vi "Auto Setup.vi"(8 "error in":errorcluster) -> (0 "error out":errorcluster)   [LabVIEW 2020]
uses:
  <vilib>/Rock Robotics/WPI/DriverStation/WPI_DriverStationRobotMode2.ctl
  b3a484b6-3d34-4235-842a-44c07264b682.vi
  19e807a5-ee4b-41d9-ac37-e9a2df102fa4.vi
  Framework/Robot Global Data.vi
  <vilib>/Rock Robotics/Network Tables/NT Write String Array.vi
  <vilib>/Rock Robotics/Network Tables/NT Write Variant.vi
  <vilib>/Rock Robotics/Network Tables/NT Read String.vi
panel:
  in  "override":bool=TRUE
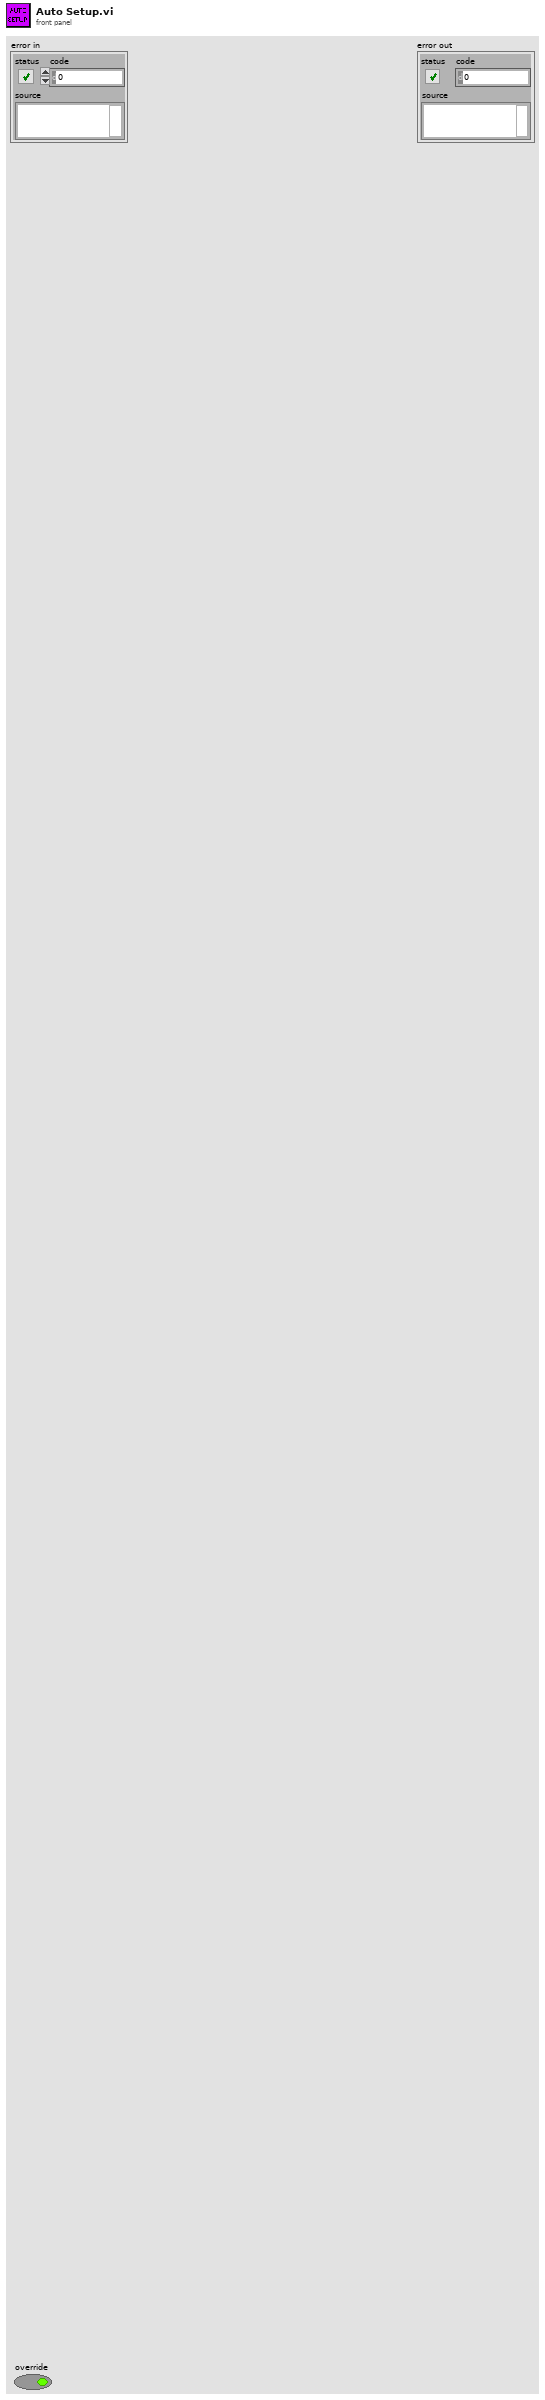
[diagram p1: front panel]
types:
  T1 = typedef "WPI_DriverStationRobotMode2.ctl" = enum16{"Autonomous Disabled", "Autonomous Enabled", "Teleop Disabled", "Teleop Enabled", "Disconnected", "Finish", "Test Disabled", "Test Enabled", "Emergency Stopped"}
  T2 = cluster{"Robot Backwards":bool, "Reverse Path":bool}
  T3 = cluster{"Segment Name":string, "Type":enum16{"Accel Straight", "Const Straight", "Blend", "Circle"}, "Traj Pos Points":cluster{"x":dbl, "y":dbl, "th":dbl}[], "Traj Vel Points":cluster{"V":dbl, "th":dbl}[], "Accel Index":i32, "Decel Index":i32}[]
  T4 = typedef "Single Cmd Info.ctl" = cluster{"Name":string, "CPTM.DataType":variant, "All Control Values Variant":cluster{"Name":string, "Variant Data":variant}[], "icon full":T5, "icon scaled":T5, "Path":path, "Subsystem Color":u32}
  T5 = typedef "imagedata.ctl" = cluster{"image type":i32, "image depth":i32, "image":u8[], "mask":u8[], "colors":u32[], "Rectangle":cluster{"left":i16, "top":i16, "right":i16, "bottom":i16}}
  T6 = typedef "Overrides.ctl" = cluster{"Count":string, "Angular Override":dbl, "Enabled?":bool, "Velocity Override":dbl, "Angle Override":dbl}[]
  T7 = typedef "Angluar Limits.ctl" = cluster{"Velocity (deg/s)":dbl, "Accel (deg/s^2)":dbl, "Jerk (deg/s^3)":dbl}
  T8 = cluster{"Sample Period (s)":dbl, cluster{"Velocity (fps)":dbl, "Accel (fps^2)":dbl, "Jerk (fps^3)":dbl, "StoopidFast (fps)":dbl}, "Conditions":cluster{"vInitial (fps)":dbl, "vFinal (fps)":dbl}, "Overrides":T6, "Angular Limits":T7}
  T9 = typedef "Drive Type.ctl" = enum16{"Nonholonomic", "Holonomic"}
  T10 = typedef "Path Type.ctl" = enum16{"Clothoid", "Bezier"}
  T11 = cluster{"Overall":cluster{"Time (s)":dbl, "Distance (ft)":dbl}, "Points out":cluster{"x":dbl, "y":dbl, "th":dbl}[], "Commands out":cluster{"Time (s)":dbl, T4, bool}[], "Zero V":bool, "Trajectory Data":cluster{"Segment Name":string, "Type":enum16{"Accel Straight", "Const Straight", "Blend", "Circle"}, "Traj Pos Points":cluster{"x":dbl, "y":dbl, "th":dbl}[], "Traj Vel Points":cluster{"V":dbl, "th":dbl}[], "Accel Index":i32, "Decel Index":i32}[], "Reversals":cluster{"Robot Backwards":bool, "Reverse Path":bool}, "Fields":cluster{"Sample Period (s)":dbl, cluster{"Velocity (fps)":dbl, "Accel (fps^2)":dbl, "Jerk (fps^3)":dbl, "StoopidFast (fps)":dbl}, "Conditions":cluster{"vInitial (fps)":dbl, "vFinal (fps)":dbl}, "Overrides":T6, "Angular Limits":T7}, "Trajectory Meta":cluster{"Drive Type":T9, "Path Type":T10}}
  T12 = cluster{"Traj Vel Points":cluster{"V":dbl, "th":dbl}[], "Reversals":cluster{"Robot Backwards":bool, "Reverse Path":bool}}
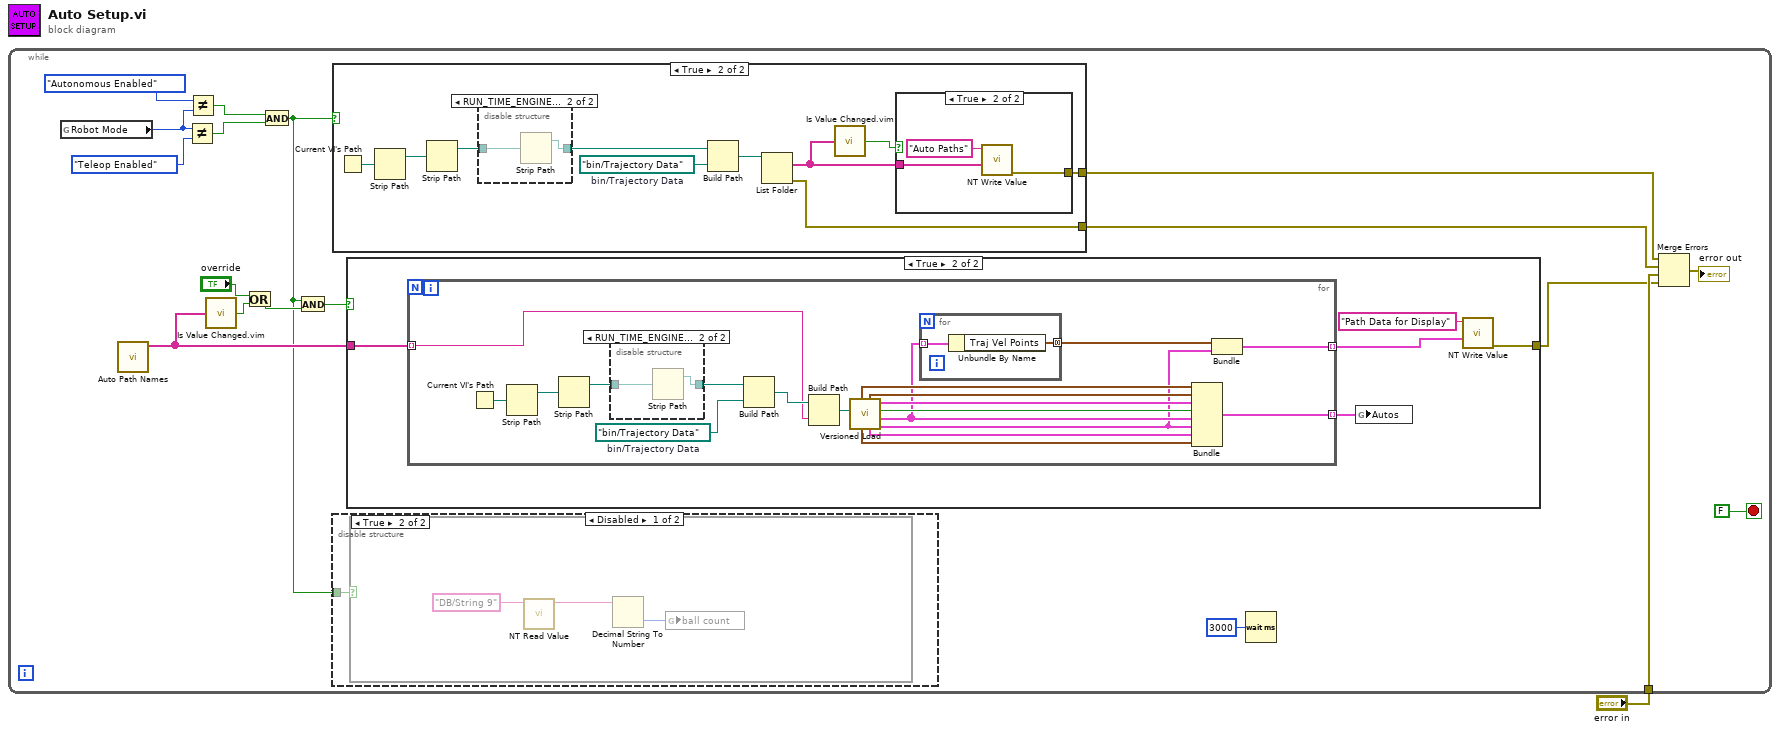
[diagram p0: block diagram]
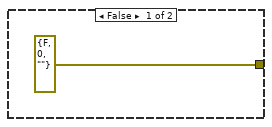
[diagram p4: hidden frame]
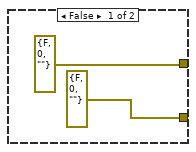
[diagram p6: hidden frame]
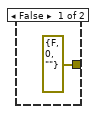
[diagram p7: hidden frame]
diagram:
  n1 = while {
    tunnel: "error in" -> [w3]
    stop <- FALSE stop-if-true
    n2 = global read "Robot Global Data.vi" "Robot Mode"() -> (w17:T1)
    n3 = call "Auto Path Names.vi"() -> ("Path Names"=w5:string[])  [unwired: 11 in]
    n4 = Not Equal?(x=w17, y=WPI_DriverStationRobotMode2."Teleop Enabled") -> (x != y?=w14:bool)
    n5 = Not Equal?(x=WPI_DriverStationRobotMode2."Autonomous Enabled", y=w17) -> (x != y?=w15:bool)
    n6 = call "Is Value Changed.vim"("value"=w5) -> ("changed or first call?"=w8:bool)
    n7 = Or(x="override", y=w8) -> (x .or. y?=w6:bool)
    n8 = And(x=w15, y=w14) -> (x .and. y?=w4:bool)
    n9 = And(x=w4, y=w6) -> (x .and. y?=w13:bool)
    n10 = case shown="True" w4 {
      tunnel: [errorcluster {"status"=FALSE, "code"=0, "source"=""} ("error out") w59] -> w12
      tunnel: [errorcluster {"status"=FALSE, "code"=0, "source"=""} ("error out") w58] -> w10
      frame False {
      }
      frame True {
        w60 = path "bin/Trajectory Data"  # bin/Trajectory Data
        n11 = Current VI's Path() -> (path=w61:path)
        n12 = Strip Path(path=w61) -> (stripped path=w62:path)  [unwired: 1 out]
        n13 = Strip Path(path=w62) -> (stripped path=w64:path)  [unwired: 1 out]
        n14 = disable-structure shown="RUN_TIME_ENGINE==True, Default" {
          disable-tunnel: [w70 w71] -> w63
          disable-tunnel: w64 -> [w70 w72]
          frame condition #0 (active) {
          }
          frame condition #1 {
            n15 = Strip Path(path=w72) -> (stripped path=w71:path)  [unwired: 1 out]
          }
        }
        n16 = Build Path(base path=w63, name or relative path=w60) -> (appended path=w65:path)
        n17 = List Folder(path=w65) -> (filenames=w57:string[], error out=w59:errorcluster)  [unwired: 3 in, 2 out]
        n18 = call "Is Value Changed.vim"("value"=w57) -> ("changed or first call?"=w56:bool)
        n19 = case shown="True" w56 {
          tunnel: w57 -> [_ w68]
          tunnel: [errorcluster {"status"=FALSE, "code"=0, "source"=""} ("error out") w67] -> w58
          frame False {
          }
          frame True {
            n20 = call-poly <vilib>:"NT Write Value.vi"("String Array"=w68, "Name"="Auto Paths") -> ("error out"=w67:errorcluster)  [unwired: 9 in]
          }
        }
      }
    }
    n21 = disable-structure shown="Disabled" {
      disable-tunnel: w4 -> [w20 _]
      frame Disabled {
        n22 = case shown="True" w20 {
          frame False {
          }
          frame True {
            n23 = call-poly <vilib>:"NT Read Value.vi"("Name"="DB/String 9") -> ("String"=w22:string)  [unwired: 9 in, 1 out]
            n24 = Decimal String To Number(string=w22) -> (number=w21:i32)  [unwired: 2 in, 1 out]
            n25 = global write "Robot Global Data.vi" "ball count"(w21) -> ()
          }
        }
      }
      frame Enabled {
      }
    }
    n26 = case shown="True" w13 {
      tunnel: w5 -> [_ w27]
      tunnel: [errorcluster {"status"=FALSE, "code"=0, "source"=""} ("error out") w28] -> w2
      frame False {
      }
      frame True {
        n27 = for {
          tunnel: w27 -> [w42] mode=indexing
          tunnel: [w41] -> w26 mode=indexing
          tunnel: [w30] -> w25 mode=indexing
          w44 = path "bin/Trajectory Data"  # bin/Trajectory Data
          n28 = Current VI's Path() -> (path=w48:path)
          n29 = Strip Path(path=w48) -> (stripped path=w47:path)  [unwired: 1 out]
          n30 = Strip Path(path=w47) -> (stripped path=w45:path)  [unwired: 1 out]
          n31 = disable-structure shown="RUN_TIME_ENGINE==True, Default" {
            disable-tunnel: [w51 w52] -> w46
            disable-tunnel: w45 -> [w51 w53]
            frame condition #0 (active) {
            }
            frame condition #1 {
              n32 = Strip Path(path=w53) -> (stripped path=w52:path)  [unwired: 1 out]
            }
          }
          n33 = Build Path(base path=w46, name or relative path=w44) -> (appended path=w43:path)
          n34 = Build Path(base path=w43, name or relative path=w42) -> (appended path=w40:path)
          n35 = call "Versioned Load.vi"("path"=w40) -> ("Reversals"=w31:T2, "Trajectory Data"=w34:T3, "Zero V"=w35:bool, "Commands out"=w36:cluster{"Time (s)":dbl, T4, bool}[], "Fields"=w33:T8, "Points out"=w37:cluster{"x":dbl, "y":dbl, "th":dbl}[], "Trajectory Meta"=w32:cluster{"Drive Type":T9, "Path Type":T10}, "Overall"=w38:cluster{"Time (s)":dbl, "Distance (ft)":dbl})  [unwired: 3 in]
          n36 = for {
            tunnel: w34 -> [w50] mode=indexing
            tunnel: [w49] -> w39 mode=concatenating
            n37 = Unbundle By Name(w50) -> ("Traj Vel Points"=w49:cluster{"V":dbl, "th":dbl}[])
          }
          n38 = Bundle("Overall"=w38, "Points out"=w37, "Commands out"=w36, "Zero V"=w35, "Trajectory Data"=w34, "Reversals"=w31, "Fields"=w33, "Trajectory Meta"=w32) -> (w30:T11)  [unwired: 1 in]
          n39 = Bundle("Traj Vel Points"=w39, "Reversals"=w31) -> (w41:T12)  [unwired: 1 in]
        }
        n40 = global write "Robot Global Data.vi" "Autos"(w25) -> ()
        n41 = call-poly <vilib>:"NT Write Value.vi"("Variant"=w26, "Name"="Path Data for Display") -> ("error out"=w28:errorcluster)  [unwired: 9 in]
      }
    }
    n42 = Wait (ms)(milliseconds to wait=u32 3000) -> ()  [unwired: 1 out]
    n43 = Merge Errors(w10, w12, w3, w2) -> (→"error out":errorcluster)
  }
